vi "Read TsQue.vi"(8 "error in (no error)":errorcluster, 11 "NiDaqMx in":refnum<class "NiDaqMx.lvclass">) -> (0 "error out":errorcluster, 2 "TsQue":refnum<queue>, 3 "NiDaqMx out":refnum<class "NiDaqMx.lvclass">)   [LabVIEW 2018, in "DigitizerPlugins.lvlib" / "NiDaqMx.lvclass"]
uses:
  NiDaqMx.lvclass
  NiDaqMx.lvclass/NiDaqMx.ctl
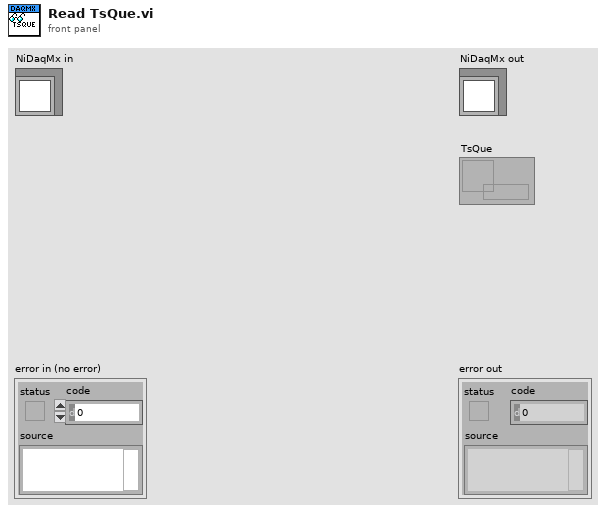
[diagram p1: front panel]
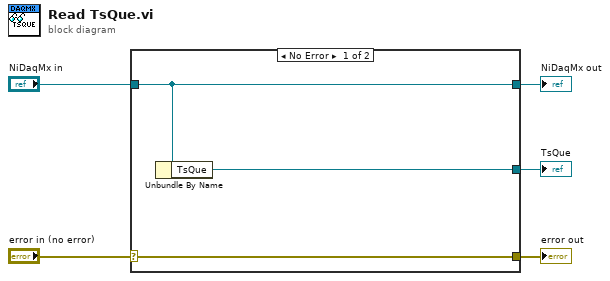
[diagram p0: block diagram]
diagram:
  n1 = case shown="No Error" "error in (no error)" {
    selector: "error in (no error)" -> [w8 w9]
    tunnel: [w8 w9] -> w4
    tunnel: [w7 w10] -> w2
    tunnel: "NiDaqMx in" -> [w7 w10]
    tunnel: [w6 _] -> w1
    frame No Error {
      n2 = Unbundle By Name(w7) -> ("TsQue"=w6:refnum<queue>)
    }
    frame Error {
    }
  }
  "error out" <- w4
  "NiDaqMx out" <- w2
  "TsQue" <- w1
